vi "Update And Broadcast Status.vi"(8 "error in (no error)":errorcluster, 10 "OK":bool, 11 "Actor in":refnum<class "Actor.lvclass">) -> (0 "error out":errorcluster, 3 "Actor out":refnum<class "Actor.lvclass">)   [LabVIEW 2015, in "Actor.lvclass"]
uses:
  Actor.lvclass
  Actor.lvclass/Actor.ctl
  Messaging/Message/Message.lvclass/Message.ctl
  Messaging/Message/Message.lvclass
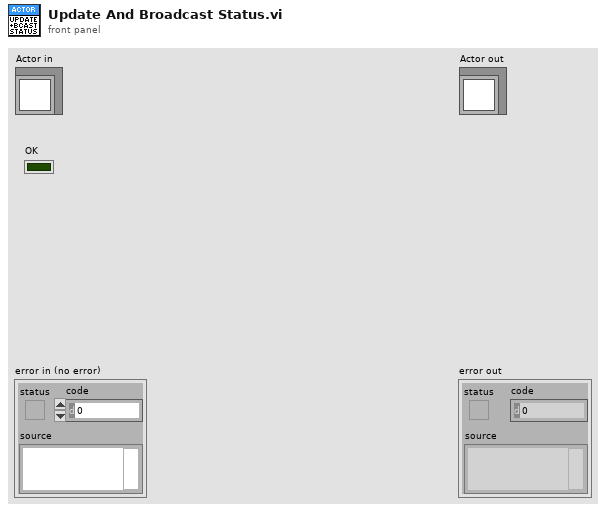
[diagram p1: front panel]
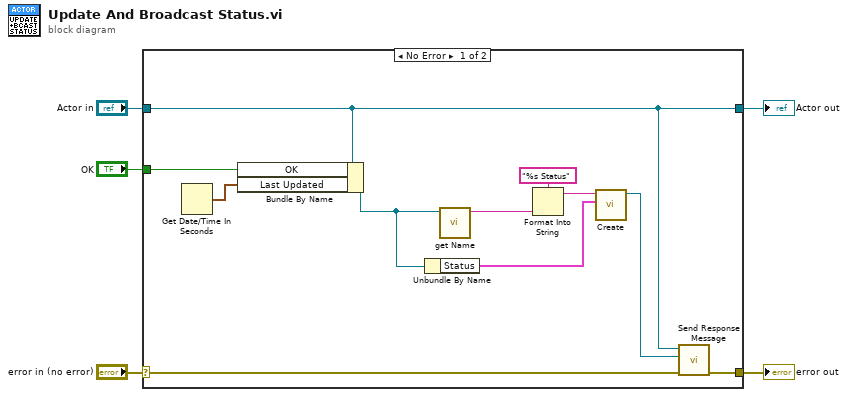
[diagram p0: block diagram]
diagram:
  n1 = case shown="No Error" "error in (no error)" {
    selector: "error in (no error)" -> [w11 w18]
    tunnel: [w10 w18] -> w4
    tunnel: [w6 w17] -> w2
    tunnel: "Actor in" -> [w6 w17]
    tunnel: "OK" -> [w16 _]
    frame No Error {
      n2 = Get Date/Time In Seconds() -> (seconds since 1Jan1904=w15:timestamp)
      n3 = Bundle By Name(cluster=w6, "OK"=w16, "Last Updated"=w15) -> (w9:refnum<class "Actor.lvclass">)
      n4 = Unbundle By Name(w9) -> ("Status"=w8:cluster{"OK":bool, "Last Updated":timestamp})
      n5 = call-dynamic "get Name.vi"("Actor in"=w9) -> ("Name"=w7:string)  [unwired: 9 in, 1 out]
      n6 = Format Into String(format string="%s Status", w7) -> (resulting string=w14:string)  [unwired: 2 in, 1 out]
      n7 = call "Create.vi"("Data"=w8, "Name"=w14) -> ("Message out"=w12:refnum<class "Message.lvclass">)  [unwired: 8 in, 1 out]
      n8 = call-dynamic "Send Response Message.vi"("error in (no error)"=w11, "Message"=w12, "Actor in"=w6) -> ("error out"=w10:errorcluster)  [unwired: 8 in]
    }
    frame Error {
    }
  }
  "error out" <- w4
  "Actor out" <- w2
